vi "cv_01-03_ReduceSamples.vi"() -> ()   [LabVIEW 2013]
panel:
  out "Table":string[][](table)
  in  "stop":bool
  out "Waveform Graph":dynamicdata(graph)
  in  "Enable":bool
  out "Mean":dbl
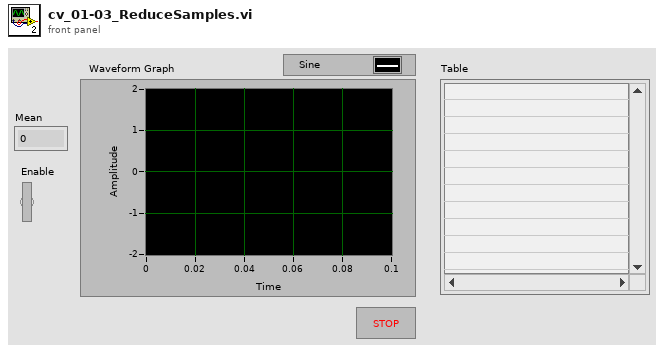
[diagram p1: front panel]
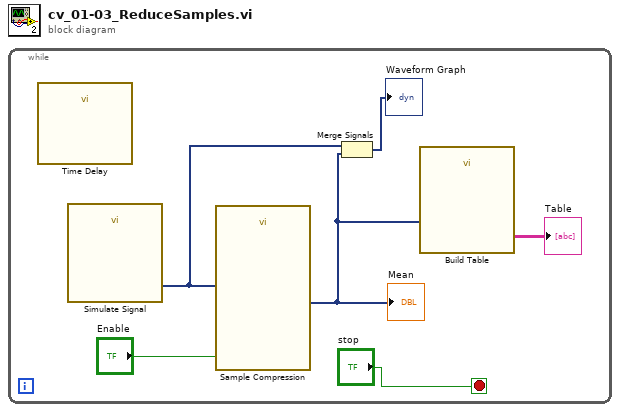
[diagram p0: block diagram]
diagram:
  n1 = while {
    stop <- "stop" stop-if-true
    n2 = call "Time Delay"() -> ()  [unwired: 11 in, 1 out]
    n3 = call "Simulate Signal"() -> ("Sine"=w5:dynamicdata)  [unwired: 14 in, 1 out]
    n4 = call "Sample Compression"("Enable"="Enable", "Signals"=w5) -> ("Mean"=w1:dynamicdata)  [unwired: 7 in, 2 out]
    "Mean" <- w1
    n5 = Merge Signals(w5, w1) -> (→"Waveform Graph":dynamicdata)
    n6 = call "Build Table"("Signals"=w1) -> ("Table"=→"Table":string[][])  [unwired: 4 in, 6 out]
  }
